vi "ProgramControlInitFP.vi"(0 "Front Panel Controls in":T1) -> (14 "Front Panel Controls out":T1)   [LabVIEW 2019, in "Universal Robot.lvclass"]
uses:
  Universal Robot.lvclass
  ProgramControlFPControls.ctl
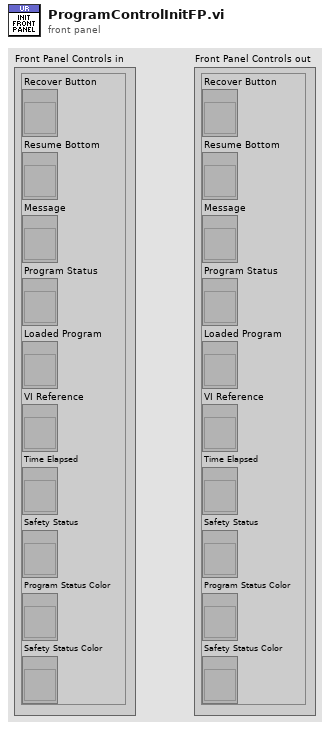
[diagram p1: front panel]
types:
  T1 = typedef "Universal Robot.lvclass/ProgramControlFPControls.ctl" = cluster{"Recover Button":refnum<vi>, "Resume Bottom":refnum<vi>, "Message":refnum<vi>, "Program Status":refnum<vi>, "Loaded Program":refnum<vi>, "VI Reference":refnum<vi>, "Time Elapsed":refnum<vi>, "Safety Status":refnum<vi>, "Program Status Color":refnum<vi>, "Safety Status Color":refnum<vi>}
  T2 = enum8{"Enabled", "Disabled", "Disabled and Grayed Out"}
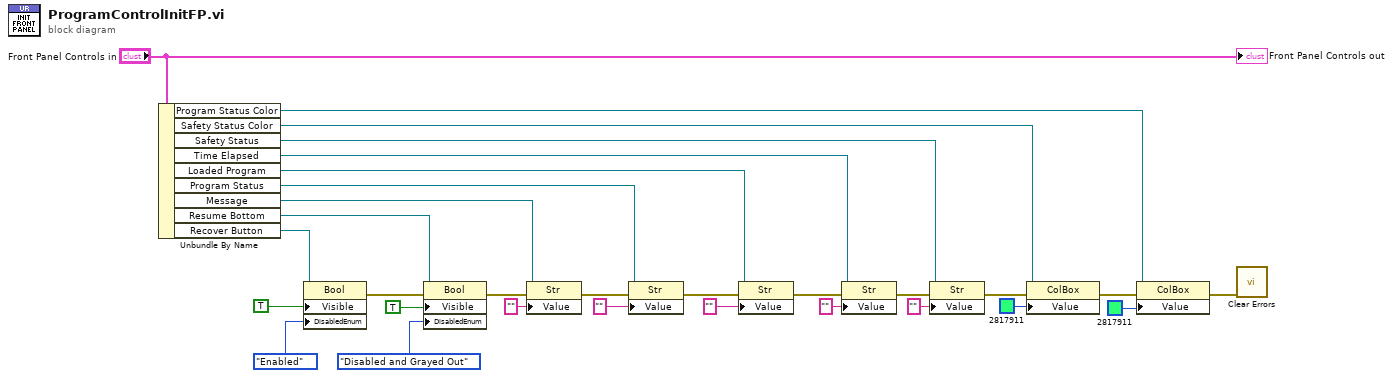
[diagram p0: block diagram]
diagram:
  n1 = Unbundle By Name("Front Panel Controls in") -> ("Program Status Color"=w4:refnum<vi>, "Safety Status Color"=w5:refnum<vi>, "Safety Status"=w9:refnum<vi>, "Time Elapsed"=w13:refnum<vi>, "Loaded Program"=w15:refnum<vi>, "Program Status"=w20:refnum<vi>, "Message"=w24:refnum<vi>, "Resume Bottom"=w26:refnum<vi>, "Recover Button"=w29:refnum<vi>)
  n2 = property class="Bool"(reference=w29, "Visible"=TRUE, "DisabledEnum"=T2."Enabled" ("Disabled")) -> (error out=w27:errorcluster)  [unwired: 1 in, 1 out]
  n3 = property class="Bool"(reference=w26, error in=w27, "Visible"=TRUE, "DisabledEnum"=T2."Disabled and Grayed Out" ("Disabled")) -> (error out=w23:errorcluster)  [unwired: 1 out]
  n4 = property class="Str"(reference=w24, error in=w23, "Value"="") -> (error out=w21:errorcluster)  [unwired: 1 out]
  n5 = property class="Str"(reference=w20, error in=w21, "Value"="") -> (error out=w16:errorcluster)  [unwired: 1 out]
  n6 = property class="Str"(reference=w15, error in=w16, "Value"="") -> (error out=w14:errorcluster)  [unwired: 1 out]
  n7 = property class="Str"(reference=w13, error in=w14, "Value"="") -> (error out=w10:errorcluster)  [unwired: 1 out]
  n8 = property class="Str"(reference=w9, error in=w10, "Value"="") -> (error out=w7:errorcluster)  [unwired: 1 out]
  n9 = property class="ColBox"(reference=w5, error in=w7, "Value"=u32 2817911) -> (error out=w8:errorcluster)  [unwired: 1 out]
  n10 = property class="ColBox"(reference=w4, error in=w8, "Value"=u32 2817911) -> (error out=w6:errorcluster)  [unwired: 1 out]
  n11 = call <vilib>:"Clear Errors.vi"("error in (no error)"=w6) -> ()  [unwired: 5 in, 2 out]
  "Front Panel Controls out" <- "Front Panel Controls in"
